vi "VFD communication.vi"() -> ()   [LabVIEW 2018]
uses:
  <vilib>/Utility/miscctls.llb/LVRectTypeDef.ctl
  <vilib>/Modbus/subvis/Modbus API/Modbus API.lvclass/Modbus API.ctl
  <vilib>/Modbus/subvis/Transmission Data Unit (ADU)/Transmission Data Unit/Transmission Data Unit.lvclass/Transmission Data Unit.ctl
  <vilib>/Modbus/master/Data Access/Unit ID/Set Unit ID Property.vi
  <vilib>/Modbus/subvis/Transmission Data Unit (ADU)/Transmission Data Unit/Data Access/Unit ID/Write Unit ID.vi
  <vilib>/Modbus/subvis/Modbus API/Read Transmission Data Unit.vi
  <vilib>/Modbus/subvis/Modbus API/Write Transmission Data Unit.vi
  <vilib>/Modbus/master/Modbus Master.lvclass
  C:/Program Files/National Instruments/LabVIEW 2018/vi.lib/Modbus/subvis/Modbus API/Modbus API.lvclass
  <vilib>/Modbus/master/Create Master Instance (TCP).vi
  <vilib>/Modbus/subvis/Transmission Data Unit (ADU)/Transmission Data Unit/Transmission Data Unit.lvclass
  <vilib>/rvi/interface/nirviOpenFPGA/nirviOpenFPGA.xnode
  <vilib>/rvi/interface/nirviMethod/nirviMethod.xnode
  <vilib>/FPGAPlugInAG/Dynamic/niLvFpga_Reset_Dynamic.vi
  <vilib>/FPGAPlugInAG/Dynamic/niLvFpga_Run_Dynamic.vi
  <vilib>/rvi/interface/nirviCloseFPGA/nirviCloseFPGA.xnode
  <vilib>/FPGAPlugInAG/Dynamic/niLvFpga_Abort_Dynamic.vi
  <vilib>/FPGAPlugInAG/Dynamic/niLvFpga_Close_Dynamic.vi
  FPGA Bitfiles/Main_FPGA_V3.lvbitx
  Main_FPGA.vi
  <vilib>/FPGAPlugInAG/cRIO-9082/niLvFpga_Open_cRIO-9082.vi
  <vilib>/rvi/interface/common/dynamic/niFpgaDynamicAddResources.vi
  <vilib>/eio/EIONode/EIONode.xnode
  <vilib>/rvi/eio/common/nirviEmuTemplateMethod_errors.vi
panel:
  in  "SPEED RPM":dbl format="%#_13g"
  in  "Brake_H":bool
  in  "Reset_H":bool
  in  "Control_H":bool
  in  "SPEED":bool
  in  "TORQUE":bool
  in  "Stop Button":bool
  out "x/y":dbl
  in  "Torque_Reference_LR 2":dbl(slide) caption="Torque \nReference" scale=-2000.0..2000.0
  out "appended array":u16[](array[numeric])
  out "*(type *) &x":i16
  out "register values":u16[](array[numeric])
  out "RPM":dbl[](array[numeric])
  in  "stop":bool
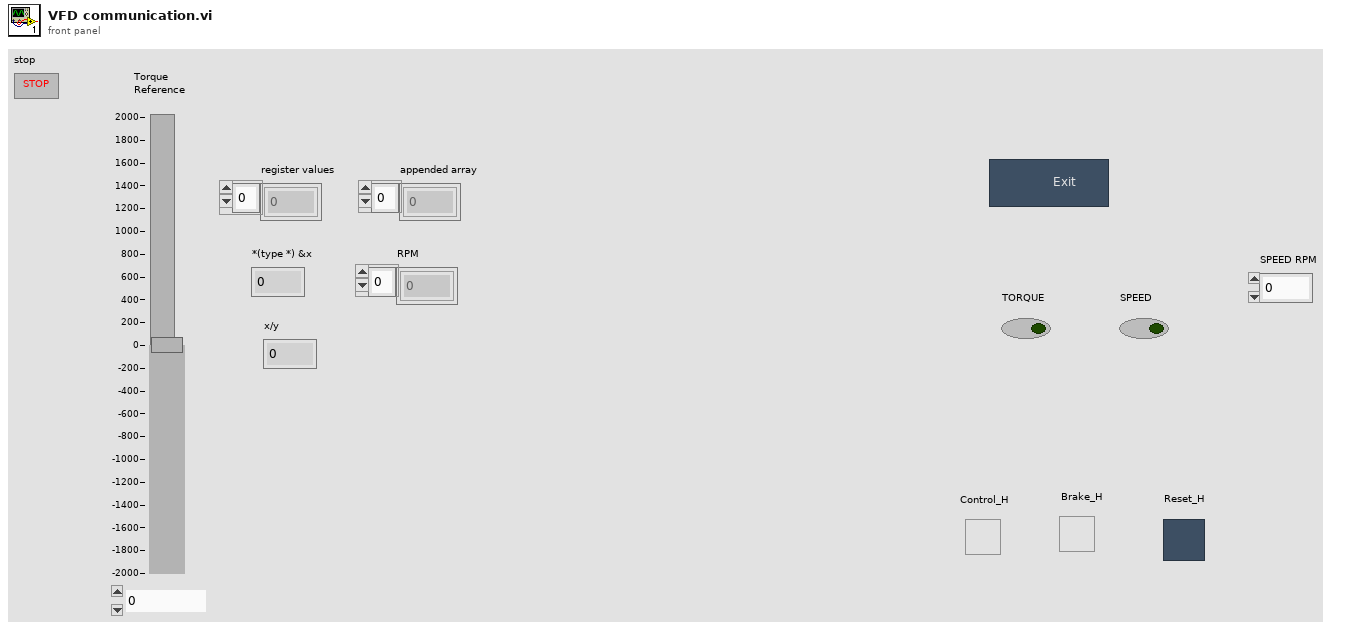
[diagram p1: front panel]
types:
  T1 = enum32{"Invalid", "Standard", "Closed", "Hidden", "Minimized", "Maximized"}
  T2 = enum32{"invalid app kind", "Development System", "Run Time System", "Student Edition", "Embedded LabVIEW", "Evaluation", "Custom"}
  T3 = typedef "LVRectTypeDef.ctl" = cluster{"Left":i16, "Top":i16, "Right":i16, "Bottom":i16}
  T4 = cluster{"Core":cluster{"Current VI Reference":refnum<vi>, "Close Panel on Exit?":bool}, "Your Boolean data":bool, "SPEED":u16[]}
  T5 = cluster{"Current VI Reference":refnum<vi>, "Close Panel on Exit?":bool}
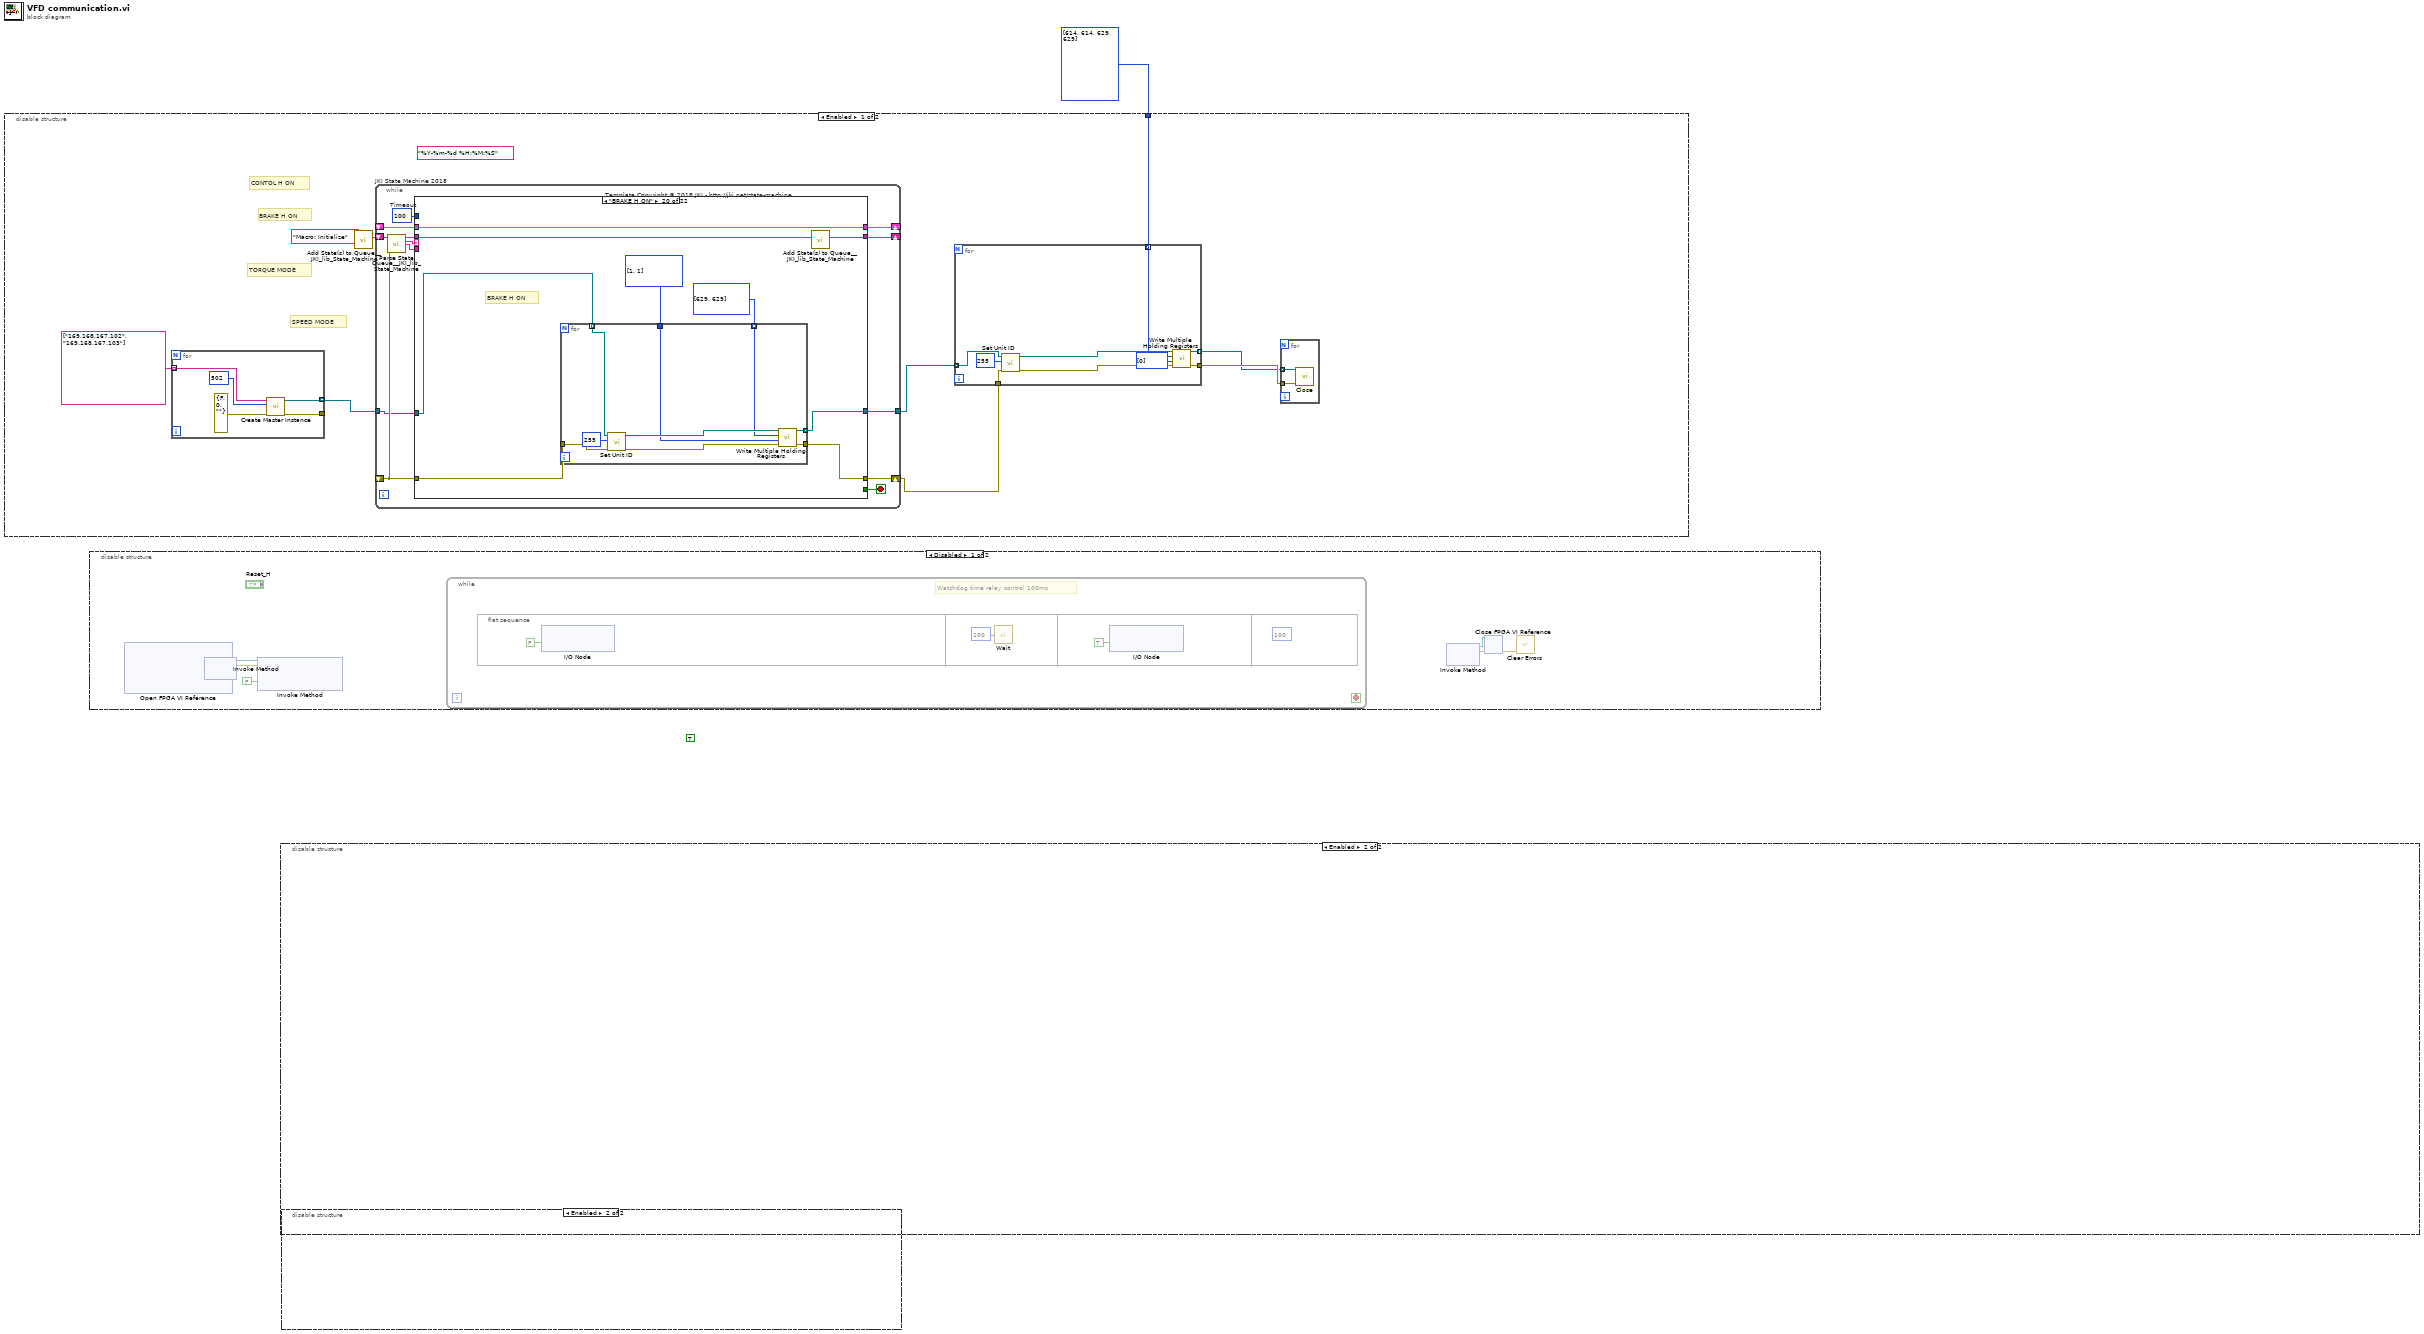
[diagram p0: block diagram]
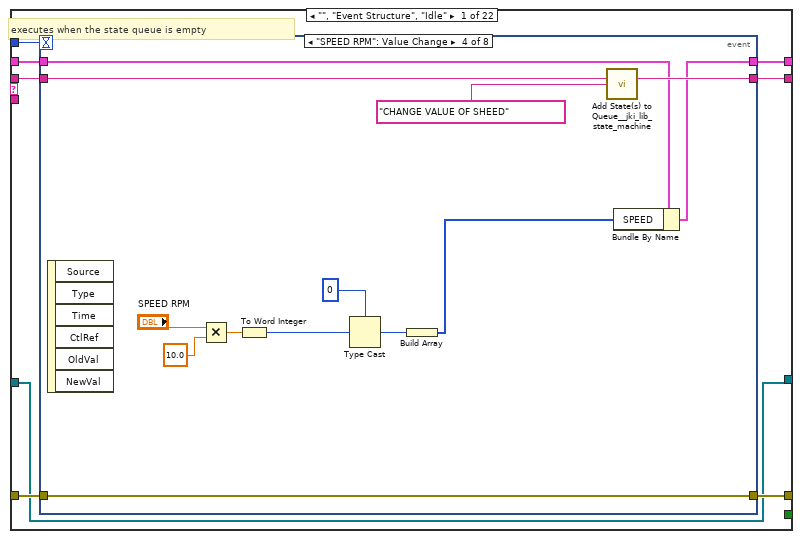
[diagram p3: hidden frame]
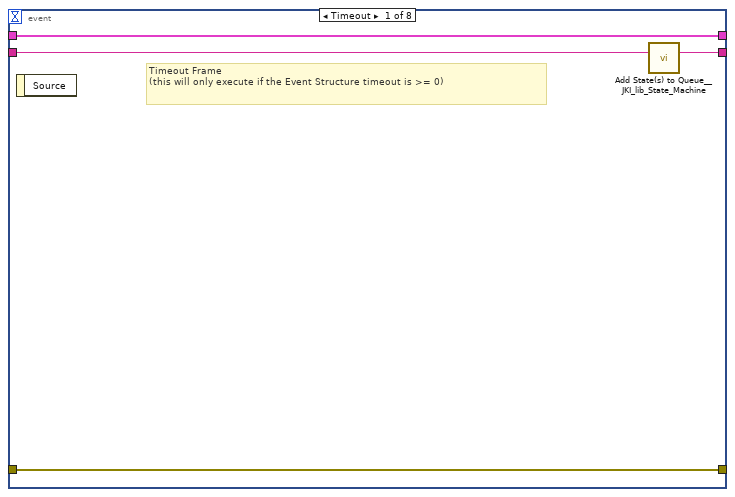
[diagram p4: hidden frame]
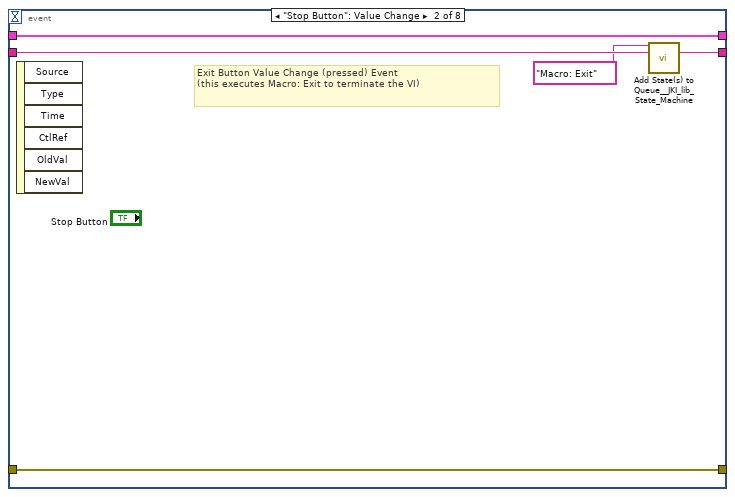
[diagram p5: hidden frame]
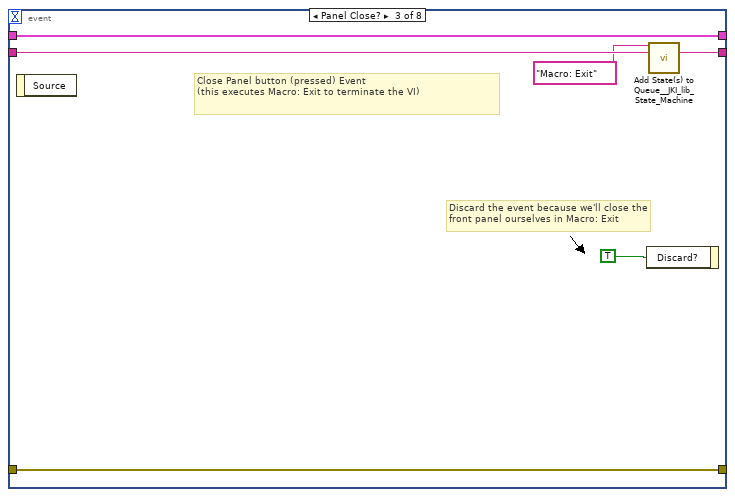
[diagram p6: hidden frame]
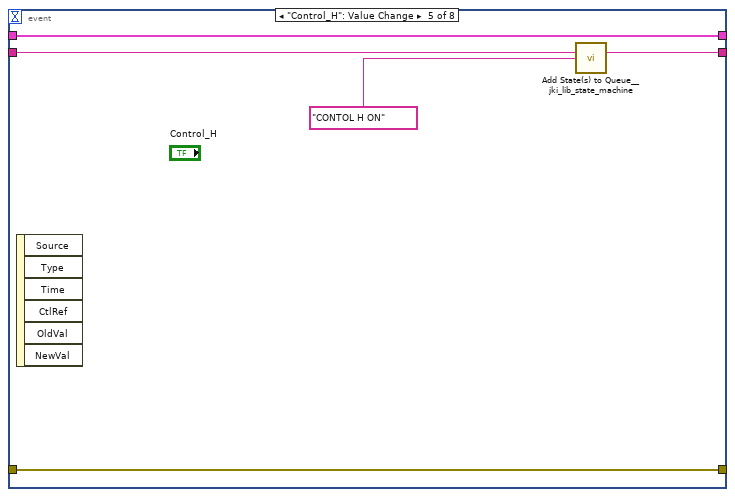
[diagram p7: hidden frame]
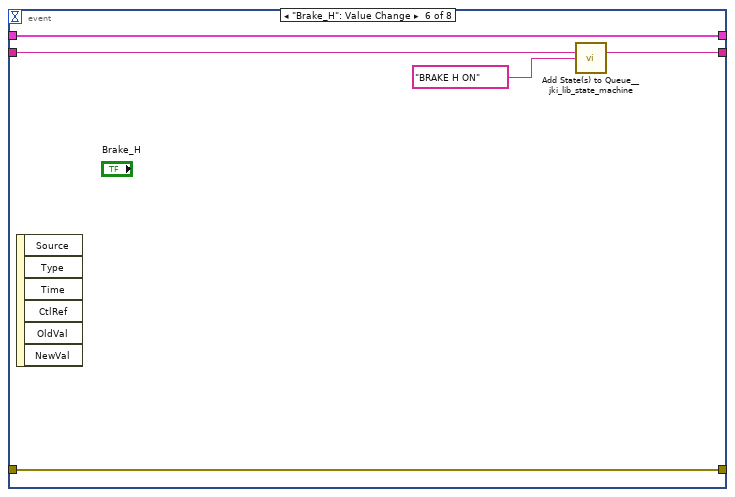
[diagram p8: hidden frame]
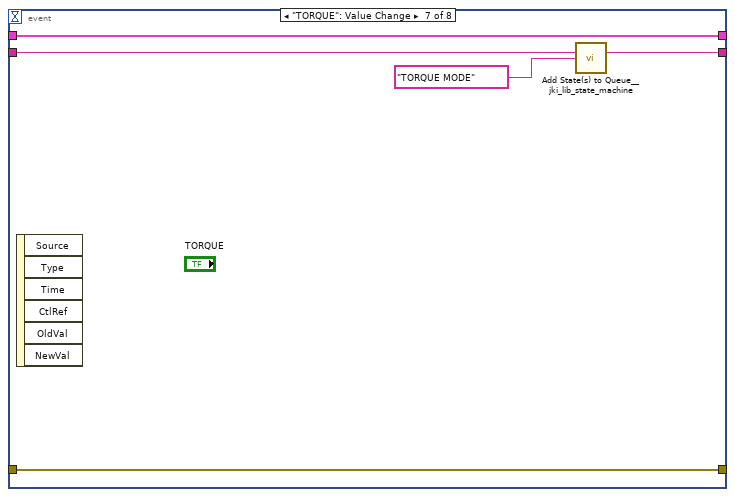
[diagram p9: hidden frame]
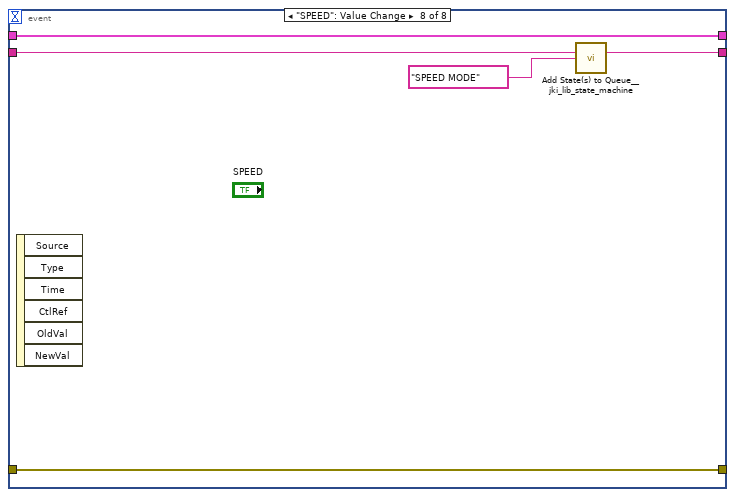
[diagram p10: hidden frame]
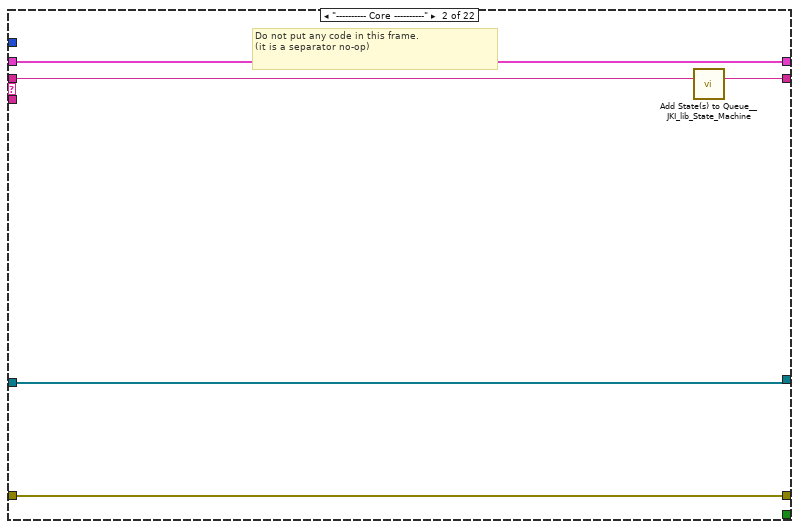
[diagram p11: hidden frame]
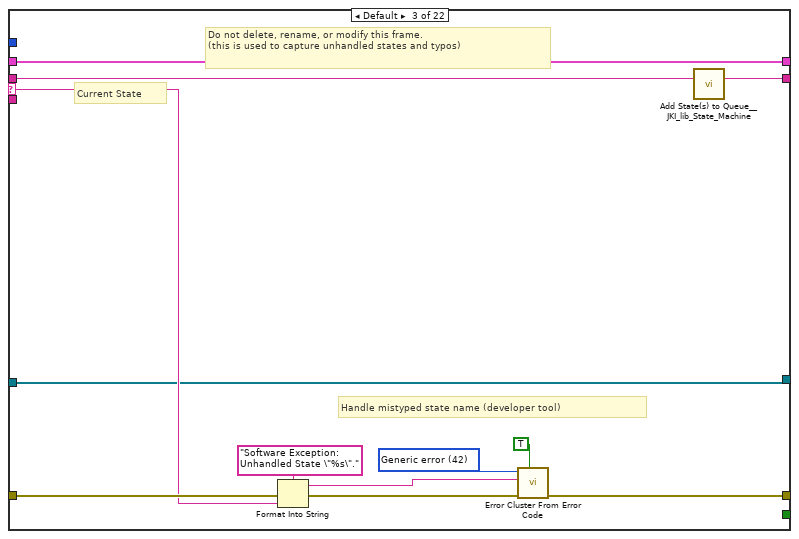
[diagram p12: hidden frame]
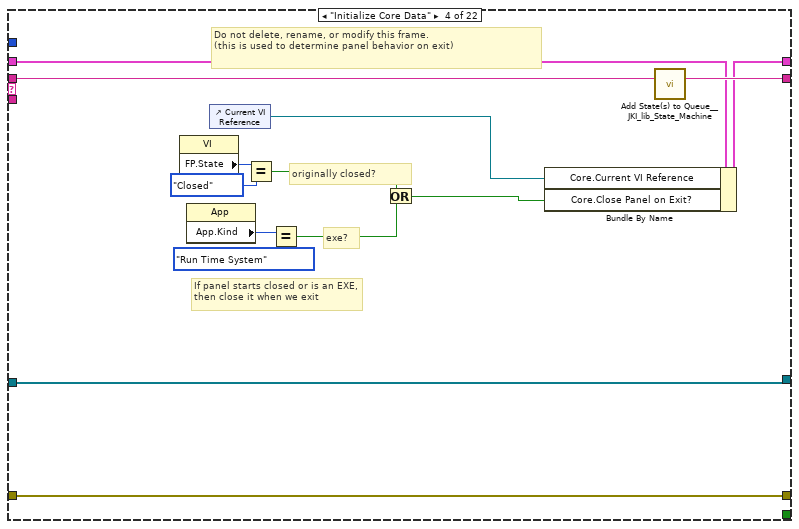
[diagram p13: hidden frame]
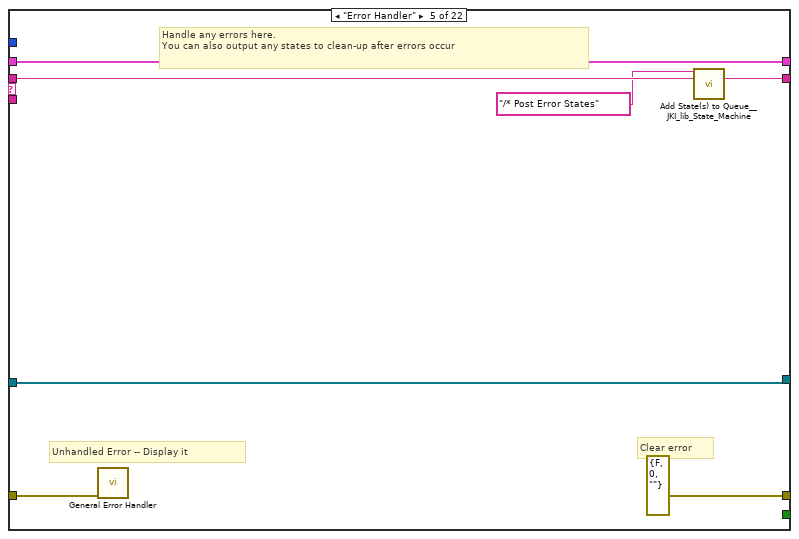
[diagram p14: hidden frame]
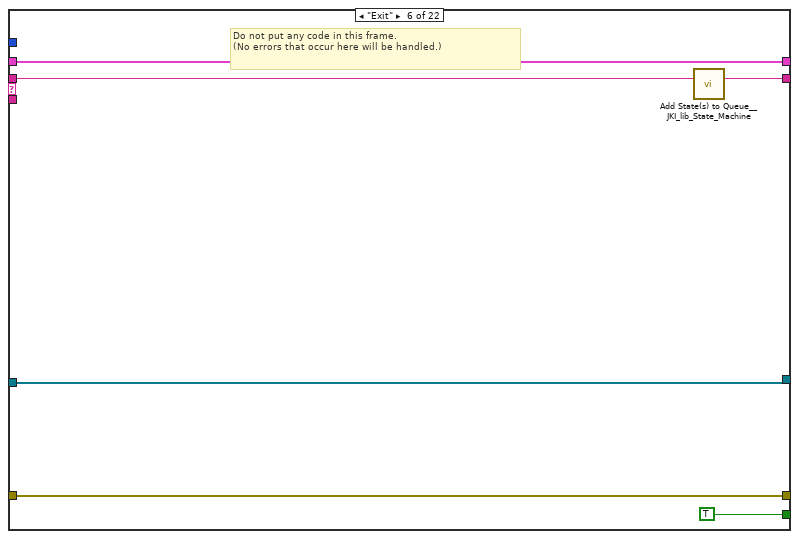
[diagram p15: hidden frame]
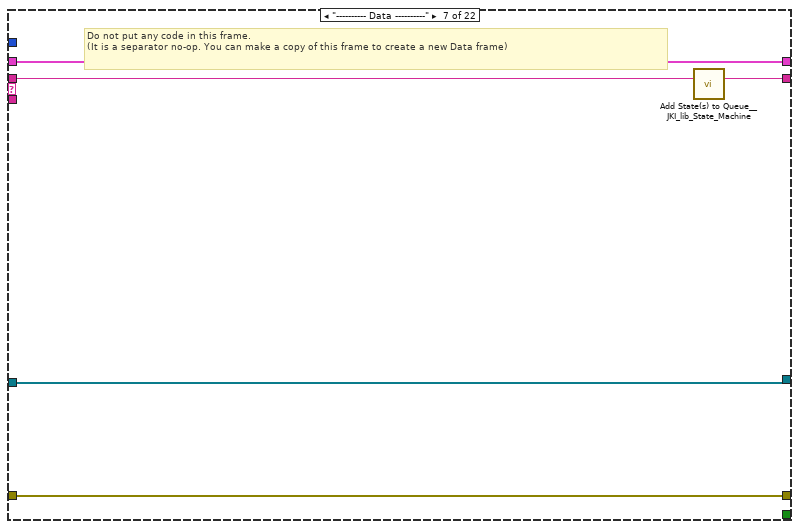
[diagram p16: hidden frame]
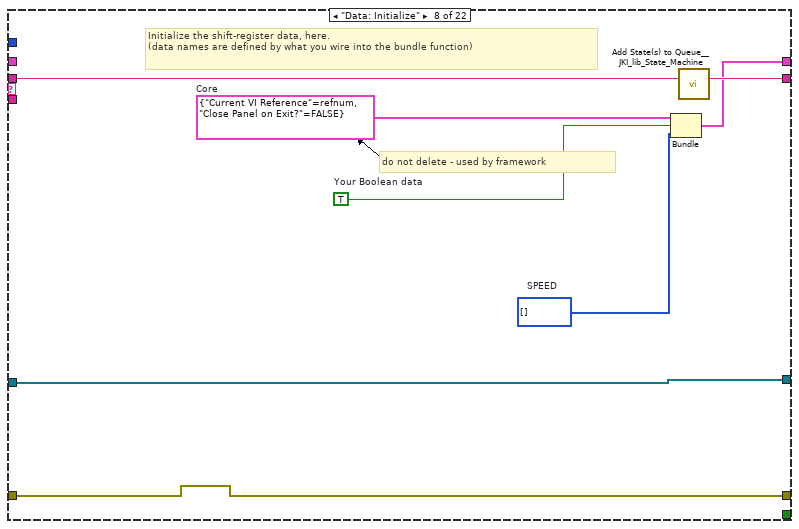
[diagram p17: hidden frame]
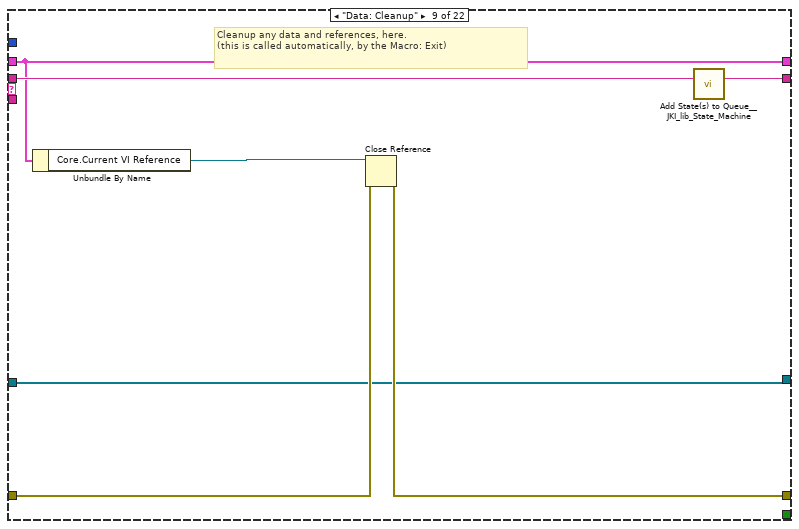
[diagram p18: hidden frame]
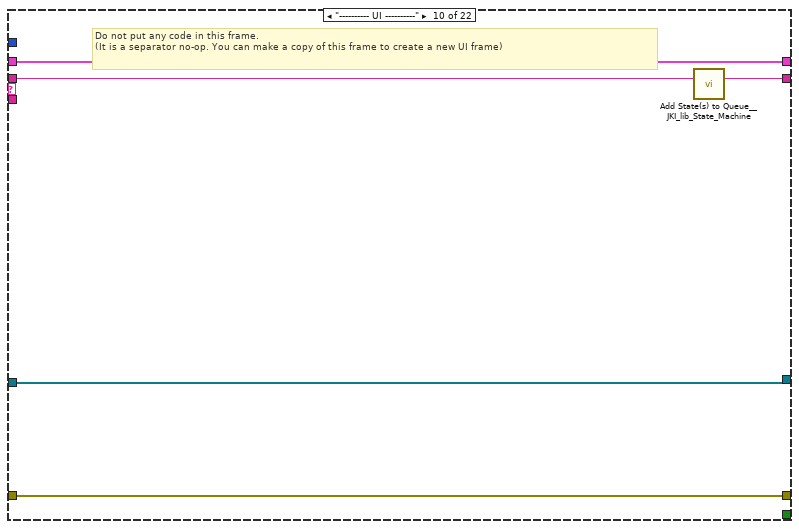
[diagram p19: hidden frame]
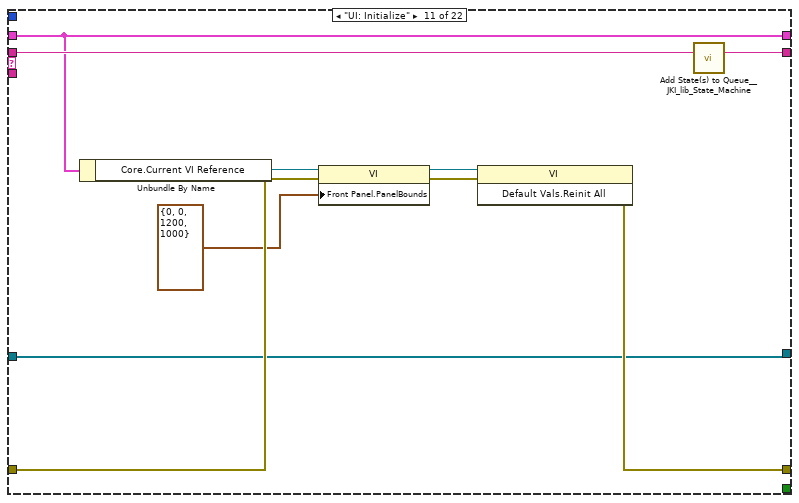
[diagram p20: hidden frame]
diagram:
  (unwired) TRUE ("Mod6/Watchdog Ready")
  n1 = disable-structure shown="Enabled" {
    disable-tunnel: u16[] [614, 614, 629, 629] ("holding register values") -> [w2 _]
    frame Enabled {
      (unwired) "%Y-%m-%d %H:%M:%S" ("time format string (%c)")
      # "SPEED MODE"
      # "TORQUE MODE"
      # "BRAKE H ON"
      # "CONTOL H ON"
      n2 = for {
        tunnel: [w24] -> _
        tunnel: string[] ["169.168.167.102", "169.168.167.103"] -> [w23] mode=indexing
        tunnel: [w22] -> w7 mode=indexing
        n3 = call-poly <vilib>:"Create Master Instance.vi"("error in (no error)"=errorcluster {"status"=FALSE, "code"=0, "source"=""}, "port (502)"=u16 502, "address"=w23) -> ("error out"=w24:errorcluster, "TCP master instance"=w22:refnum<class "Modbus Master.lvclass">)  [unwired: 7 in]
      }
      n4 = call <vilib>:"Add State(s) to Queue__JKI_lib_State_Machine.vi"("State(s) in (\"\")"="Macro: Initialize") -> ("States Out"=w10:string)  [unwired: 14 in]
      n5 = while "JKI State Machine 2018" {
        shift-right: [w32] -> _
        shift-left: _ -> [w31]
        shift-right: [w35] -> w5
        shift-left: _ -> [w29]
        shift-right: [w34] -> _
        shift-left: w10 -> [w36]
        tunnel: w7 -> [w28]
        tunnel: [w27] -> w6
        stop <- w33 stop-if-true
        w30 = 100  # Timeout
        # "Template Copyright © 2018 JKI - http://jki.net/state-machine"
        n6 = call <vilib>:"Parse State Queue__JKI_lib_State_Machine.vi"("State Queue"=w36, "Error In (no error)"=w29) -> ("Remaining States"=w38:string, "Current State"=w39:string, "Arguments"=w37:string)  [unwired: 11 in]
        n7 = case shown="\"BRAKE H ON\"" w39 {
          selector: w39 -> [_ _ w102 _ _ _ _ _ _ _ _ _ _ _ _ _ _ _ _ _ _ _]
          tunnel: w38 -> [w47 w100 w106 w126 w133 w139 w144 w152 w159 w164 w174 w181 w193 w263 w269 w280 w285 w294 w312 w330 w348 w366]
          tunnel: w37 -> [_ _ _ _ _ _ _ _ _ _ _ w176 w187 _ _ _ _ _ _ _ _ _]
          tunnel: w31 -> [w45 w97 w104 w119 w130 w137 w141 _ w154 w161 w172 w179 w189 w260 w266 w277 w282 w292 w310 w328 w346 w364]
          tunnel: [w44 w98 w108 w123 errorcluster {"status"=FALSE, "code"=0, "source"=""} ("error out") w136 w142 w147 w155 w162 w166 w177 w190 w261 w267 w278 w283 w290 w308 w326 w344 w362] -> w35
          tunnel: w29 -> [w43 w98 w107 w123 w129 w136 w142 w147 w156 w162 w170 w178 w191 w261 w267 w278 w283 w291 w309 w327 w345 w363]
          tunnel: [w46 w99 w105 w125 w132 w138 w143 w151 w158 w163 w173 w180 w192 w262 w268 w279 w284 w293 w311 w329 w347 w365] -> w34
          tunnel: [_ _ _ _ _ TRUE _ _ _ _ _ _ _ _ _ _ _ _ _ _ _ _] -> w33
          tunnel: [w42 w97 w104 w124 w130 w137 w141 w150 w154 w161 w172 w179 w189 w260 w266 w277 w282 w292 w310 w328 w346 w364] -> w32
          tunnel: w30 -> [w41 _ _ _ _ _ _ _ _ _ _ _ _ _ _ _ _ _ _ _ _ _]
          tunnel: [w40 w96 w101 w113 w127 w134 w140 w146 w153 w160 w165 w175 w186 w259 w264 w270 w281 w288 w304 w322 w340 w358] -> w27
          tunnel: w28 -> [w40 w96 w101 w113 w127 w134 w140 w146 w153 w160 w165 w175 w186 w259 w264 w270 w281 w289 w307 w325 w343 w361]
          frame "", "Event Structure", "Idle" {
            # "executes when the state queue is empty"
            n8 = event shown="[3] \"SPEED RPM\": Value Change" {
              selector: _ -> [_ _ _ _ _ _ _ _]
              dyn-events: _ -> [_ _ _ _ _ _ _ _]
              timeout: w41 -> [_ _ _ _ _ _ _ _]
              tunnel: w47 -> [w51 w56 w62 w73 w77 w82 w87 w92]
              tunnel: [w50 w55 w61 w74 w78 w83 w88 w93] -> w46
              tunnel: w45 -> [w48 w53 w59 w65 w79 w84 w89 w94]
              tunnel: [w49 w54 w60 w75 w80 w85 w90 w95] -> w44
              tunnel: w43 -> [w49 w54 w60 w75 w80 w85 w90 w95]
              tunnel: [w48 w53 w59 w63 w79 w84 w89 w94] -> w42
              event Timeout {
                # "Timeout Frame\n(this will only execute if the Event Structure timeout is >= 0)"
                n9 = event-data() -> ()  [unwired: 1 in, 1 out]
                n10 = call <vilib>:"Add State(s) to Queue__JKI_lib_State_Machine.vi"("State(s) in (\"\")"=w51) -> ("States Out"=w50:string)  [unwired: 14 in]
              }
              event "Stop Button": Value Change {
                # "Exit Button Value Change (pressed) Event\n(this executes Macro: Exit to terminate the VI)"
                n11 = event-data() -> ()  [unwired: 1 in, 6 out]
                n12 = call <vilib>:"Add State(s) to Queue__JKI_lib_State_Machine.vi"("State(s) in Front (\"\")"="Macro: Exit", "State(s) in (\"\")"=w56) -> ("States Out"=w55:string)  [unwired: 13 in]
              }
              event Panel Close? {
                # "Discard the event because we'll close the front panel ourselves in Macro: Exit"
                # "Close Panel button (pressed) Event\n(this executes Macro: Exit to terminate the VI)"
                n13 = event-data() -> ()  [unwired: 1 in, 1 out]
                n14 = event-data("Discard?"=TRUE) -> ()  [unwired: 1 in, 1 out]
                n15 = call <vilib>:"Add State(s) to Queue__JKI_lib_State_Machine.vi"("State(s) in Front (\"\")"="Macro: Exit", "State(s) in (\"\")"=w62) -> ("States Out"=w61:string)  [unwired: 13 in]
              }
              event "SPEED RPM": Value Change {
                n16 = event-data() -> ()  [unwired: 1 in, 6 out]
                n17 = Multiply(x="SPEED RPM", y=10.0) -> (x*y=w68:dbl)
                n18 = To Word Integer(number=w68) -> (16bit integer=w70:i16)
                n19 = Type Cast(type=u16 0, x=w70) -> (*(type *) &x=w69:u16)
                n20 = Build Array(w69) -> (w64:u16[])
                n21 = call <vilib>:"Add State(s) to Queue__jki_lib_state_machine.vi"("State(s) in (\"\")"=w73, "State(s) at Back (\"\")"="CHANGE VALUE OF SHEED" ("State(s) at Back (\"\")")) -> ("States Out"=w74:string)  [unwired: 13 in]
                n22 = Bundle By Name(cluster=w65, "SPEED"=w64) -> (w63:T4)
              }
              event "Control_H": Value Change {
                n23 = event-data() -> ()  [unwired: 1 in, 6 out]
                n24 = call <vilib>:"Add State(s) to Queue__jki_lib_state_machine.vi"("State(s) in (\"\")"=w77, "State(s) at Back (\"\")"="CONTOL H ON" ("State(s) at Back (\"\")")) -> ("States Out"=w78:string)  [unwired: 13 in]
              }
              event "Brake_H": Value Change {
                n25 = event-data() -> ()  [unwired: 1 in, 6 out]
                n26 = call <vilib>:"Add State(s) to Queue__jki_lib_state_machine.vi"("State(s) in (\"\")"=w82, "State(s) at Back (\"\")"="BRAKE H ON" ("State(s) at Back (\"\")")) -> ("States Out"=w83:string)  [unwired: 13 in]
              }
              event "TORQUE": Value Change {
                n27 = event-data() -> ()  [unwired: 1 in, 6 out]
                n28 = call <vilib>:"Add State(s) to Queue__jki_lib_state_machine.vi"("State(s) in (\"\")"=w87, "State(s) at Back (\"\")"="TORQUE MODE" ("State(s) at Back (\"\")")) -> ("States Out"=w88:string)  [unwired: 13 in]
              }
              event "SPEED": Value Change {
                n29 = event-data() -> ()  [unwired: 1 in, 6 out]
                n30 = call <vilib>:"Add State(s) to Queue__jki_lib_state_machine.vi"("State(s) in (\"\")"=w92, "State(s) at Back (\"\")"="SPEED MODE" ("State(s) at Back (\"\")")) -> ("States Out"=w93:string)  [unwired: 13 in]
              }
            }
          }
          frame "---------- Core ----------" {
            # "Do not put any code in this frame.\n(it is a separator no-op)"
            n31 = call <vilib>:"Add State(s) to Queue__JKI_lib_State_Machine.vi"("State(s) in (\"\")"=w100) -> ("States Out"=w99:string)  [unwired: 14 in]
          }
          frame Default {
            w111 = 42 items=["No error", "Argument error", "Memory is full", "Out of zone", "End of file", "File already open", "Generic file I/O error", "File not found", "File permission error", "Disk is full", "Duplicate path", "Too many files open", "System feature not enabled", "Resource file not found", "Cannot add resource", "Resource not found", "Image not found", "Image memory error", "Pen does not exist", "Config type invalid", "Config token not found", "Config parse error", "Config memory error", "Bad external code format", "Bad external code offset", "External code not present", "Null window", "Destroy window error", "Null menu", "Print aborted", "Bad print record", "Print driver error", "Windows error during printing", "Memory error during printing", "Print dialog error", "Generic print error", "Invalid device refnum", "Device not found", "Device parameter error", "Device unit error", "Cannot open device", "Device call aborted", "Generic error", "Cancelled by user", "Object ID too low", "Object ID too high", "Object not in heap", "Unknown heap", "Unknown object (invalid DefProc)", "Unknown object (DefProc not in table)", "Message out of range", "Invalid (null) method", "Unknown message", "Manager call not supported", "Bad address", "Network operation in progress", "Network operation timed out", "Connection is busy", "Network attribute not supported", "Network error", "Address in use", "System out of memory", "Connection aborted", "Connection refused", "Not connected", "Already connected", "Connection closed", "Initialization error (interapplication manager)", "Bad occurrence", "Wait on unbound occurrence handler", "Occurrence queue overflow", "Datalog type conflict", "Unused", "Unrecognized type (interapplication manager)", "Memory corrupt", "Failed to make temporary DLL", "Old CIN version", "Drag socket not found", "Failed to load drop-object", "Failed to register OLE object", "Failed to release OLE object", "Format specifier type mismatch", "Unknown format specifier", "Too few format specifiers", "Too many format specifiers", "Scan failed", "Newer CIN version", "Error converting to variant", "Runtime menu error", "Password tampered", "Variant attribute not found", "Incompatible variant data type", "Event data is not available", "Event Store is not present", "Occurrence is not found", "Event Queue is not created", "Event info is not available", "Refnum passed is NULL", "Error retrieving Class GUID", "Error retrieving CoClass GUID", "Error retrieving TypeLib GUID.", "Bad built application magic bytes.", "Specific driver is different from the specific driver associated with the Logical Name.", "There is no session opened to the class driver.", "Max Error", "MAX - Error with config objects", "MAX - Error loading configuration", "MAX - Group not supported"]
            # "Current State"
            # "Do not delete, rename, or modify this frame.\n(this is used to capture unhandled states and typos)"
            # "Handle mistyped state name (developer tool)"
            n32 = Format Into String(format string="Software Exception: Unhandled State \"%s\"." ("message"), error in=w107, w102) -> (resulting string=w110:string, error out=w109:errorcluster)  [unwired: 1 in]
            n33 = call <vilib>:"Error Cluster From Error Code.vi"("show call chain? (False)"=TRUE, "error in (no error)"=w109, "error message (\"\")"=w110, "error code (0)"=w111) -> ("error out"=w108:errorcluster)  [unwired: 5 in]
            n34 = call <vilib>:"Add State(s) to Queue__JKI_lib_State_Machine.vi"("State(s) in (\"\")"=w106) -> ("States Out"=w105:string)  [unwired: 14 in]
          }
          frame "Initialize Core Data" {
            # "Do not delete, rename, or modify this frame.\n(this is used to determine panel behavior on exit)"
            # "originally closed?"
            # "exe?"
            # "If panel starts closed or is an EXE, then close it when we exit"
            n35 = property class="VI"() -> ("FP.State"=w116:T1)  [unwired: 2 in, 2 out]
            n36 = property class="App"() -> ("App.Kind"=w122:T2)  [unwired: 2 in, 2 out]
            n37 = control-ref of="Current VI Reference"() -> (w117:refnum<vi>)
            n38 = Equal?(x=w116, y=T1."Closed" ("Front Panel Window:State")) -> (x = y?=w114:bool)
            n39 = Equal?(x=w122, y=T2."Run Time System" ("Application:Kind")) -> (x = y?=w120:bool)
            n40 = Or(x=w114, y=w120) -> (x .or. y?=w118:bool)
            n41 = Bundle By Name(cluster=w119, "Core.Current VI Reference"=w117, "Core.Close Panel on Exit?"=w118) -> (w124:T4)
            n42 = call <vilib>:"Add State(s) to Queue__JKI_lib_State_Machine.vi"("State(s) in (\"\")"=w126) -> ("States Out"=w125:string)  [unwired: 14 in]
          }
          frame "Error Handler" {
            # "Unhandled Error -- Display it"
            # "Handle any errors here.\nYou can also output any states to clean-up after errors occur"
            # "Clear error"
            n43 = call <vilib>:"General Error Handler.vi"("error in (no error)"=w129) -> ()  [unwired: 10 in, 5 out]
            n44 = call <vilib>:"Add State(s) to Queue__JKI_lib_State_Machine.vi"("State(s) in Front (\"\")"="/* Post Error States", "State(s) in (\"\")"=w133) -> ("States Out"=w132:string)  [unwired: 13 in]
          }
          frame "Exit" {
            # "Do not put any code in this frame.\n(No errors that occur here will be handled.)"
            n45 = call <vilib>:"Add State(s) to Queue__JKI_lib_State_Machine.vi"("State(s) in (\"\")"=w139) -> ("States Out"=w138:string)  [unwired: 14 in]
          }
          frame "---------- Data ----------" {
            # "Do not put any code in this frame.\n(It is a separator no-op. You can make a copy of this frame to create a new Data frame)"
            n46 = call <vilib>:"Add State(s) to Queue__JKI_lib_State_Machine.vi"("State(s) in (\"\")"=w144) -> ("States Out"=w143:string)  [unwired: 14 in]
          }
          frame "Data: Initialize" {
            w145 = u16[] []  # SPEED
            w148 = T5 {"Current VI Reference"=refnum, "Close Panel on Exit?"=FALSE}  # Core
            w149 = TRUE  # Your Boolean data
            # "do not delete - used by framework"
            # "Initialize the shift-register data, here.\n(data names are defined by what you wire into the bundle function)"
            n47 = Bundle("Core"=w148, "Your Boolean data"=w149, "SPEED"=w145) -> (w150:T4)  [unwired: 1 in]
            n48 = call <vilib>:"Add State(s) to Queue__JKI_lib_State_Machine.vi"("State(s) in (\"\")"=w152) -> ("States Out"=w151:string)  [unwired: 14 in]
          }
          frame "Data: Cleanup" {
            # "Cleanup any data and references, here.\n(this is called automatically, by the Macro: Exit)"
            n49 = Unbundle By Name(w154) -> ("Core.Current VI Reference"=w157:refnum<vi>)
            n50 = Close Reference(reference=w157, error in (no error)=w156) -> (error out=w155:errorcluster)
            n51 = call <vilib>:"Add State(s) to Queue__JKI_lib_State_Machine.vi"("State(s) in (\"\")"=w159) -> ("States Out"=w158:string)  [unwired: 14 in]
          }
          frame "---------- UI ----------" {
            # "Do not put any code in this frame.\n(It is a separator no-op. You can make a copy of this frame to create a new UI frame)"
            n52 = call <vilib>:"Add State(s) to Queue__JKI_lib_State_Machine.vi"("State(s) in (\"\")"=w164) -> ("States Out"=w163:string)  [unwired: 14 in]
          }
          frame "UI: Initialize" {
            n53 = Unbundle By Name(w172) -> ("Core.Current VI Reference"=w171:refnum<vi>)
            n54 = property class="VI"(reference=w171, error in=w170, "Front Panel.PanelBounds"=T3 {"Left"=0, "Top"=0, "Right"=1200, "Bottom"=1000} ("Front Panel Window:Panel Bounds")) -> (reference out=w168:refnum<vi>, error out=w167:errorcluster)
            n55 = invoke class="VI" method="Default Vals.Reinit All"(reference=w168, error in=w167) -> (error out=w166:errorcluster)  [unwired: 1 in, 2 out]
            n56 = call <vilib>:"Add State(s) to Queue__JKI_lib_State_Machine.vi"("State(s) in (\"\")"=w174) -> ("States Out"=w173:string)  [unwired: 14 in]
          }
          frame "UI: Cursor Set" {
            # "Argument"
            # "Set and Unset Cursor Busy.\n(Usage: \"UI: Cursor Set >> Busy|Idle\")"
            n57 = case shown="\"Idle\", Default" w176 {
              tunnel: w178 -> [w183 w185]
              tunnel: [w182 w184] -> w177
              frame "Idle", Default {
                n58 = call <vilib>:"Unset Busy.vi"("error in (no error)"=w183) -> ("error out"=w182:errorcluster)  [unwired: 10 in]
              }
              frame "Busy" {
                n59 = call <vilib>:"Set Busy.vi"("error in (no error)"=w185) -> ("error out"=w184:errorcluster)  [unwired: 9 in, 1 out]
              }
            }
            n60 = call <vilib>:"Add State(s) to Queue__JKI_lib_State_Machine.vi"("State(s) in (\"\")"=w181) -> ("States Out"=w180:string)  [unwired: 14 in]
          }
          frame "UI: Front Panel State" {
            # "Argument"
            # "Set Front Panel Open or Closed\n(Usage: \"UI: Front Panel State >> Open|Close\")"
            n61 = Unbundle By Name(w189) -> ("Core.Current VI Reference"=w188:refnum<vi>)
            n62 = case shown="\"Minimize\", \"Minimized\"" w187 {
              tunnel: w191 -> [w199 w214 w225 w238 w251]
              tunnel: [w201 w215 w227 w240 w253] -> w190
              tunnel: w188 -> [w200 w212 w226 w239 w252]
              frame "Open", "Standard", Default {
                w194 = T1."Standard" ("State")
                n63 = property class="VI"(reference=w200, error in=w199) -> (reference out=w197:refnum<vi>, error out=w198:errorcluster, "FP.State"=w196:T1)
                n64 = Not Equal?(x=w196, y=w194) -> (x != y?=w195:bool)
                n65 = case shown="True" w195 {
                  tunnel: [w205 w207] -> w201
                  tunnel: w198 -> [w204 w207]
                  tunnel: w197 -> [w203 _]
                  tunnel: w194 -> [w202 _]
                  frame True {
                    n66 = invoke class="VI" method="FP.Open"(reference=w203, error in=w204, "Activate"=TRUE, "State"=w202) -> (error out=w205:errorcluster)  [unwired: 1 in, 4 out]
                  }
                  frame False {
                  }
                }
              }
              frame "Close", "Closed" {
                n67 = property class="VI"(reference=w212, error in=w214) -> (reference out=w211:refnum<vi>, error out=w213:errorcluster, "FP.State"=w209:T1)
                n68 = Not Equal?(x=w209, y=T1."Closed" ("Front Panel Window:State")) -> (x != y?=w208:bool)
                n69 = case shown="True" w208 {
                  tunnel: [w216 w219] -> w215
                  tunnel: w213 -> [w216 w218]
                  tunnel: w211 -> [_ w217]
                  frame False {
                  }
                  frame True {
                    n70 = invoke class="VI" method="FP.Close"(reference=w217, error in=w218) -> (error out=w219:errorcluster)  [unwired: 1 in, 2 out]
                  }
                }
              }
              frame "Hidden", "Hide" {
                w220 = T1."Hidden" ("State")
                n71 = property class="VI"(reference=w226, error in=w225) -> (reference out=w223:refnum<vi>, error out=w224:errorcluster, "FP.State"=w222:T1)
                n72 = Not Equal?(x=w222, y=w220) -> (x != y?=w221:bool)
                n73 = case shown="True" w221 {
                  tunnel: [w231 w232] -> w227
                  tunnel: w224 -> [w230 w232]
                  tunnel: w223 -> [w229 _]
                  tunnel: w220 -> [w228 _]
                  frame True {
                    n74 = invoke class="VI" method="FP.Open"(reference=w229, error in=w230, "State"=w228) -> (error out=w231:errorcluster)  [unwired: 2 in, 4 out]
                  }
                  frame False {
                  }
                }
              }
              frame "Minimize", "Minimized" {
                w233 = T1."Minimized" ("State")
                n75 = property class="VI"(reference=w239, error in=w238) -> (reference out=w236:refnum<vi>, error out=w237:errorcluster, "FP.State"=w235:T1)
                n76 = Not Equal?(x=w235, y=w233) -> (x != y?=w234:bool)
                n77 = case shown="True" w234 {
                  tunnel: [w244 w245] -> w240
                  tunnel: w237 -> [w243 w245]
                  tunnel: w236 -> [w242 _]
                  tunnel: w233 -> [w241 _]
                  frame True {
                    n78 = invoke class="VI" method="FP.Open"(reference=w242, error in=w243, "State"=w241) -> (error out=w244:errorcluster)  [unwired: 2 in, 4 out]
                  }
                  frame False {
                  }
                }
              }
              frame "Maximize", "Maximized" {
                w246 = T1."Maximized" ("State")
                n79 = property class="VI"(reference=w252, error in=w251) -> (reference out=w249:refnum<vi>, error out=w250:errorcluster, "FP.State"=w248:T1)
                n80 = Not Equal?(x=w248, y=w246) -> (x != y?=w247:bool)
                n81 = case shown="True" w247 {
                  tunnel: [w257 w258] -> w253
                  tunnel: w250 -> [w256 w258]
                  tunnel: w249 -> [w255 _]
                  tunnel: w246 -> [w254 _]
                  frame True {
                    n82 = invoke class="VI" method="FP.Open"(reference=w255, error in=w256, "State"=w254) -> (error out=w257:errorcluster)  [unwired: 2 in, 4 out]
                  }
                  frame False {
                  }
                }
              }
            }
            n83 = call <vilib>:"Add State(s) to Queue__JKI_lib_State_Machine.vi"("State(s) in (\"\")"=w193) -> ("States Out"=w192:string)  [unwired: 14 in]
          }
          frame "---------- Macro ----------" {
            # "Do not put any code in this frame.\n(It is a separator no-op. You can make a copy of this frame to create a new Macro frame)"
            n84 = call <vilib>:"Add State(s) to Queue__JKI_lib_State_Machine.vi"("State(s) in (\"\")"=w263) -> ("States Out"=w262:string)  [unwired: 14 in]
          }
          frame "Macro: Initialize" {
            w265 = "Data: Initialize\nInitialize Core Data\nUI: Initialize\nUI: Front Panel State >> Open"  # Data: Initialize Initialize Core Data UI: Initialize UI: Front Panel State >> Open
            # "Initialization Macro\n(This is called once, when the VI starts)"
            n85 = call <vilib>:"Add State(s) to Queue__JKI_lib_State_Machine.vi"("State(s) in Front (\"\")"=w265, "State(s) in (\"\")"=w269) -> ("States Out"=w268:string)  [unwired: 13 in]
          }
          frame "Macro: Exit" {
            # "Exit Macro\n(This is called once, when the VI exits)"
            n86 = Unbundle By Name(w277) -> ("Core.Close Panel on Exit?"=w276:bool)
            n87 = Select(t="UI: Front Panel State >> Close", s=w276, f="") -> (s? t:f=w273:string)
            n88 = call <vilib>:"Add State(s) to Queue__JKI_lib_State_Machine.vi"("State(s) in (\"\")"=w273, "State(s) at Back (\"\")"="Data: Cleanup\nExit") -> ("States Out"=w271:string)  [unwired: 13 in]
            n89 = call <vilib>:"Add State(s) to Queue__JKI_lib_State_Machine.vi"("State(s) in Front (\"\")"=w271, "State(s) in (\"\")"=w280) -> ("States Out"=w279:string)  [unwired: 13 in]
          }
          frame "---------- New Category ----------" {
            # "Template Separator\n(You can make a copy of, or modify, this frame)"
            n90 = call <vilib>:"Add State(s) to Queue__JKI_lib_State_Machine.vi"("State(s) in (\"\")"=w285) -> ("States Out"=w284:string)  [unwired: 14 in]
          }
          frame "CHANGE VALUE OF SHEED" {
            w287 = u16[] [121, 121]  # address
            n91 = Unbundle By Name(w292) -> ("SPEED"=w286:u16[])
            n92 = for {
              tunnel: w291 -> [w298]
              tunnel: w289 -> [w300] mode=indexing
              tunnel: [w303] -> w288 mode=indexing
              tunnel: [w302] -> w290
              tunnel: w287 -> [w296] mode=indexing
              tunnel: w286 -> [w295]
              n93 = call <vilib>:"Set Unit ID.vi"("error in (no error)"=w298, "unit ID"=u8 255, "Modbus master in"=w300) -> ("error out"=w297:errorcluster, "Modbus master out"=w299:refnum<class "Modbus Master.lvclass">)  [unwired: 7 in]
              n94 = call-dynamic "Write Multiple Holding Registers.vi"("error in (no error)"=w297, "holding register values"=w295, "starting address"=w296, "Modbus master in"=w299) -> ("error out"=w302:errorcluster, "Modbus master out"=w303:refnum<class "Modbus Master.lvclass">)  [unwired: 6 in]
            }
            n95 = call <vilib>:"Add State(s) to Queue__JKI_lib_State_Machine.vi"("State(s) in (\"\")"=w294) -> ("States Out"=w293:string)  [unwired: 14 in]
          }
          frame "CONTOL H ON" {
            # "CONTOL H ON"
            n96 = for {
              tunnel: w307 -> [w315] mode=indexing
              tunnel: w309 -> [w317]
              tunnel: [w321] -> w304 mode=indexing
              tunnel: [w320] -> w308
              tunnel: u16[] [1, 1] ("holding register values") -> [w314]
              tunnel: u16[] [614, 614] ("holding register values") -> [w313] mode=indexing
              n97 = call <vilib>:"Set Unit ID.vi"("error in (no error)"=w317, "unit ID"=u8 255, "Modbus master in"=w315) -> ("error out"=w316:errorcluster, "Modbus master out"=w318:refnum<class "Modbus Master.lvclass">)  [unwired: 7 in]
              n98 = call-dynamic "Write Multiple Holding Registers.vi"("error in (no error)"=w316, "holding register values"=w314, "starting address"=w313, "Modbus master in"=w318) -> ("error out"=w320:errorcluster, "Modbus master out"=w321:refnum<class "Modbus Master.lvclass">)  [unwired: 6 in]
            }
            n99 = call <vilib>:"Add State(s) to Queue__JKI_lib_State_Machine.vi"("State(s) in (\"\")"=w312) -> ("States Out"=w311:string)  [unwired: 14 in]
          }
          frame "BRAKE H ON" {
            # "BRAKE H ON"
            n100 = for {
              tunnel: w325 -> [w333] mode=indexing
              tunnel: w327 -> [w335]
              tunnel: [w339] -> w322 mode=indexing
              tunnel: [w338] -> w326
              tunnel: u16[] [1, 1] ("holding register values") -> [w332]
              tunnel: u16[] [629, 629] ("holding register values") -> [w331] mode=indexing
              n101 = call <vilib>:"Set Unit ID.vi"("error in (no error)"=w335, "unit ID"=u8 255, "Modbus master in"=w333) -> ("error out"=w334:errorcluster, "Modbus master out"=w336:refnum<class "Modbus Master.lvclass">)  [unwired: 7 in]
              n102 = call-dynamic "Write Multiple Holding Registers.vi"("error in (no error)"=w334, "holding register values"=w332, "starting address"=w331, "Modbus master in"=w336) -> ("error out"=w338:errorcluster, "Modbus master out"=w339:refnum<class "Modbus Master.lvclass">)  [unwired: 6 in]
            }
            n103 = call <vilib>:"Add State(s) to Queue__JKI_lib_State_Machine.vi"("State(s) in (\"\")"=w330) -> ("States Out"=w329:string)  [unwired: 14 in]
          }
          frame "TORQUE MODE" {
            # "TORQUE MODE"
            n104 = for {
              tunnel: w343 -> [w351] mode=indexing
              tunnel: w345 -> [w353]
              tunnel: [w357] -> w340 mode=indexing
              tunnel: [w356] -> w344
              tunnel: u16[] [1] ("holding register values") -> [w350]
              tunnel: u16[] [1835] ("holding register values") -> [w349] mode=indexing
              n105 = call <vilib>:"Set Unit ID.vi"("error in (no error)"=w353, "unit ID"=u8 255, "Modbus master in"=w351) -> ("error out"=w352:errorcluster, "Modbus master out"=w354:refnum<class "Modbus Master.lvclass">)  [unwired: 7 in]
              n106 = call-dynamic "Write Multiple Holding Registers.vi"("error in (no error)"=w352, "holding register values"=w350, "starting address"=w349, "Modbus master in"=w354) -> ("error out"=w356:errorcluster, "Modbus master out"=w357:refnum<class "Modbus Master.lvclass">)  [unwired: 6 in]
            }
            n107 = call <vilib>:"Add State(s) to Queue__JKI_lib_State_Machine.vi"("State(s) in (\"\")"=w348) -> ("States Out"=w347:string)  [unwired: 14 in]
          }
          frame "SPEED MODE" {
            # "SPEED MODE"
            n108 = for {
              tunnel: w361 -> [w369] mode=indexing
              tunnel: w363 -> [w371]
              tunnel: [w375] -> w358 mode=indexing
              tunnel: [w374] -> w362
              tunnel: u16[] [1] ("holding register values") -> [w368]
              tunnel: u16[] [1835] ("holding register values") -> [w367] mode=indexing
              n109 = call <vilib>:"Set Unit ID.vi"("error in (no error)"=w371, "unit ID"=u8 255, "Modbus master in"=w369) -> ("error out"=w370:errorcluster, "Modbus master out"=w372:refnum<class "Modbus Master.lvclass">)  [unwired: 7 in]
              n110 = call-dynamic "Write Multiple Holding Registers.vi"("error in (no error)"=w370, "holding register values"=w368, "starting address"=w367, "Modbus master in"=w372) -> ("error out"=w374:errorcluster, "Modbus master out"=w375:refnum<class "Modbus Master.lvclass">)  [unwired: 6 in]
            }
            n111 = call <vilib>:"Add State(s) to Queue__JKI_lib_State_Machine.vi"("State(s) in (\"\")"=w366) -> ("States Out"=w365:string)  [unwired: 14 in]
          }
        }
      }
      n112 = for {
        tunnel: w6 -> [w13] mode=indexing
        tunnel: [w19] -> w3 mode=indexing
        tunnel: [w18] -> w4
        tunnel: w2 -> [w14] mode=indexing
        tunnel: w5 -> [w12]
        n113 = call <vilib>:"Set Unit ID.vi"("error in (no error)"=w12, "unit ID"=u8 255, "Modbus master in"=w13) -> ("error out"=w15:errorcluster, "Modbus master out"=w16:refnum<class "Modbus Master.lvclass">)  [unwired: 7 in]
        n114 = call-dynamic "Write Multiple Holding Registers.vi"("error in (no error)"=w15, "holding register values"=u16[] [0], "starting address"=w14, "Modbus master in"=w16) -> ("error out"=w18:errorcluster, "Modbus master out"=w19:refnum<class "Modbus Master.lvclass">)  [unwired: 6 in]
      }
      n115 = for {
        tunnel: w4 -> [w21]
        tunnel: w3 -> [w20] mode=indexing
        n116 = call-dynamic "Close.vi"("error in (no error)"=w21, "Modbus master in"=w20) -> ()  [unwired: 9 in, 1 out]
      }
    }
    frame Disabled {
    }
  }
  n117 = disable-structure shown="Disabled" {
    frame Disabled {
      n118 = xnode "Open FPGA VI Reference"() -> ("FPGA VI Reference Out"=w383:refnum<k20>, "error out"=w382:errorcluster)  [unwired: 2 in]
      n119 = xnode "Invoke Method"("FPGA VI Reference In"=w383, "error in"=w382) -> ("FPGA VI Reference Out"=w381:refnum<k20>, "error out"=w380:errorcluster)
      n120 = xnode "Invoke Method"("FPGA VI Reference In"=w381, "error in"=w380, "Wait Until Done (F)"=FALSE) -> ()  [unwired: 2 out]
      n121 = while {
        stop <- _ stop-if-true
        # "Watchdog time relay control 100ms"
        n122 = flat-sequence {
          frame #0 {
            n123 = xnode "I/O Node"("Mod4/DO16"=FALSE) -> ()  [unwired: 1 in, 1 out]
          }
          frame #1 {
            n124 = call "Wait"("Count(mSec)"=u32 100) -> ()  [unwired: 1 out]
          }
          frame #2 {
            n125 = xnode "I/O Node"("Mod4/DO16"=TRUE) -> ()  [unwired: 1 in, 1 out]
          }
          frame #3 {
            (unwired) u32 100 ("Count(mSec)")
          }
        }
      }
      n126 = xnode "Invoke Method"() -> ("FPGA VI Reference Out"=w378:refnum<k20>, "error out"=w377:errorcluster)  [unwired: 2 in]
      n127 = xnode "Close FPGA VI Reference"("FPGA VI Reference In"=w378, "error in"=w377) -> ("error out"=w376:errorcluster)
      n128 = call <vilib>:"Clear Errors.vi"("error in (no error)"=w376) -> ()  [unwired: 5 in, 2 out]
    }
    frame Enabled {
    }
  }
  n129 = disable-structure shown="Enabled" {
    frame Disabled {
      (unwired) 0.0 ("x/y")
      w392 = u16[] [408, 408]  # address
      (unwired) u16[] [146, 146]  # address
      w398 = u16[] [146, 146]  # address
      n130 = for {
        tunnel: [w469] -> w396
        tunnel: string[] ["169.168.167.102", "169.168.167.103"] -> [w468] mode=indexing
        tunnel: [w467] -> w401 mode=indexing
        n131 = call-poly <vilib>:"Create Master Instance.vi"("error in (no error)"=errorcluster {"status"=FALSE, "code"=0, "source"=""}, "port (502)"=u16 502, "address"=w468) -> ("error out"=w469:errorcluster, "TCP master instance"=w467:refnum<class "Modbus Master.lvclass">)  [unwired: 7 in]
      }
      n132 = Divide(x="Torque_Reference_LR 2", y=20.0) -> (x/y=w387:dbl)
      "x/y" <- w387
      n133 = Multiply(x=w387, y=10.0) -> (x*y=w391:dbl)
      n134 = To Word Integer(number=w391) -> (16bit integer=w399:i16)
      n135 = Type Cast(type=u16 0, x=w399) -> (*(type *) &x=w397:u16)
      n136 = Build Array(w397) -> (w393:u16[])
      "appended array" <- w393
      n137 = disable-structure shown="Disabled" {
        disable-tunnel: w401 -> [w410 w421]
        disable-tunnel: w398 -> [w409 _]
        disable-tunnel: w396 -> [w408 w420]
        disable-tunnel: [w407 w421] -> w395
        disable-tunnel: [w406 w420] -> w394
        disable-tunnel: w393 -> [w405 _]
        frame Disabled {
          n138 = for {
            tunnel: w410 -> [w414] mode=indexing
            tunnel: w405 -> [_] mode=indexing
            tunnel: w409 -> [w419] mode=indexing
            tunnel: w408 -> [w412]
            tunnel: [w417] -> w407 mode=indexing
            tunnel: [w416] -> w406 mode=indexing
            n139 = call <vilib>:"Set Unit ID.vi"("error in (no error)"=w412, "unit ID"=u8 255, "Modbus master in"=w414) -> ("error out"=w411:errorcluster, "Modbus master out"=w413:refnum<class "Modbus Master.lvclass">)  [unwired: 7 in]
            n140 = call-dynamic "Write Multiple Holding Registers.vi"("error in (no error)"=w411, "holding register values"=u16[] [1], "starting address"=w419, "Modbus master in"=w413) -> ("error out"=w416:errorcluster, "Modbus master out"=w417:refnum<class "Modbus Master.lvclass">)  [unwired: 6 in]
          }
        }
        frame Enabled {
        }
      }
      n141 = disable-structure shown="Enabled" {
        disable-tunnel: [w423 w452] -> w404
        disable-tunnel: [w422 w453] -> w402
        disable-tunnel: w395 -> [_ w454]
        disable-tunnel: w394 -> [_ w455]
        disable-tunnel: w393 -> [_ w450]
        disable-tunnel: w392 -> [_ w451]
        frame Disabled {
          n142 = while {
            shift-right: [w427] -> w423
            shift-left: _ -> [w428]
            shift-right: [w426] -> w422
            shift-left: _ -> [w429]
            stop <- "stop" stop-if-true
            n143 = for {
              shift-right: [w444] -> w427
              shift-left: w428 -> [w448]
              tunnel: [w443] -> w426 mode=indexing
              tunnel: [w435] -> w425 mode=indexing
              tunnel: w429 -> [w433] mode=indexing
              tunnel: [w432] -> w424
              w434 = u16 301  # starting address
              w439 = i16 0  # I16
              w445 = u16 1  # NHR
              n144 = call <vilib>:"Set Unit ID.vi"("error in (no error)"=w448, "unit ID"=u8 255, "Modbus master in"=w433) -> ("error out"=w446:errorcluster, "Modbus master out"=w447:refnum<class "Modbus Master.lvclass">)  [unwired: 7 in]
              n145 = call-dynamic "Read Holding Registers.vi"("error in (no error)"=w446, "number of holding registers"=w445, "starting address"=w434, "Modbus master in"=w447) -> ("error out"=w444:errorcluster, "register values"=w442:u16[], "Modbus master out"=w443:refnum<class "Modbus Master.lvclass">)  [unwired: 5 in]
              "register values" <- w442
              n146 = Index Array(array=w442, index=0) -> (element=w440:u16)
              n147 = Type Cast(type=w439, x=w440) -> (*(type *) &x=w432:i16)
              n148 = To Double Precision Float(number=w432) -> (double precision float=w438:dbl)
              n149 = Divide(x=w438, y=10.0) -> (x/y=w436:dbl)
              n150 = Absolute Value(x=w436) -> (abs(x)=w435:dbl)
            }
            "RPM" <- w425
            "*(type *) &x" <- w424
            n151 = Wait (ms)(milliseconds to wait=u32 5) -> ()  [unwired: 1 out]
          }
        }
        frame Enabled {
          n152 = for {
            tunnel: w455 -> [w457]
            tunnel: w454 -> [w459] mode=indexing
            tunnel: [w464] -> w453 mode=indexing
            tunnel: [w463] -> w452 mode=indexing
            tunnel: w451 -> [w462] mode=indexing
            tunnel: w450 -> [w461]
            (unwired) u16[] [22] ("holding register values")
            n153 = call <vilib>:"Set Unit ID.vi"("error in (no error)"=w457, "unit ID"=u8 255, "Modbus master in"=w459) -> ("error out"=w456:errorcluster, "Modbus master out"=w458:refnum<class "Modbus Master.lvclass">)  [unwired: 7 in]
            n154 = call-dynamic "Write Multiple Holding Registers.vi"("error in (no error)"=w456, "holding register values"=w461, "starting address"=w462, "Modbus master in"=w458) -> ("error out"=w463:errorcluster, "Modbus master out"=w464:refnum<class "Modbus Master.lvclass">)  [unwired: 6 in]
          }
        }
      }
      n155 = for {
        tunnel: w404 -> [w466] mode=indexing
        tunnel: w402 -> [w465] mode=indexing
        n156 = call-dynamic "Close.vi"("error in (no error)"=w466, "Modbus master in"=w465) -> ()  [unwired: 9 in, 1 out]
      }
    }
    frame Enabled {
    }
  }
  n157 = disable-structure shown="Enabled" {
    frame Disabled {
      n158 = To Long Integer(number=10.0) -> (32bit integer=w479:i32)
      n159 = Split Number(x=w479) -> (hi(x)=w478:u16, lo(x)=w477:u16)
      n160 = Build Array(w477, w478) -> (w476:u16[])
      n161 = call-poly <vilib>:"Create Master Instance.vi"("error in (no error)"=errorcluster {"status"=FALSE, "code"=0, "source"=""}, "port (502)"=u16 502, "address"="169.168.167.102") -> ("error out"=w475:errorcluster, "TCP master instance"=w484:refnum<class "Modbus Master.lvclass">)  [unwired: 7 in]
      n162 = for {
        tunnel: w476 -> [w491] mode=indexing
        tunnel: [w490] -> w472 mode=indexing
        tunnel: [w489] -> w474
        tunnel: w475 -> [w489]
        tunnel: u8 0 -> [w488]
        n163 = Type Cast(type=w488, x=w491) -> (*(type *) &x=w490:u8)
      }
      n164 = call-dynamic "Write Multiple Holding Registers.vi"("error in (no error)"=w474, "holding register values"=w472, "starting address"=u16 135, "Modbus master in"=w484) -> ("error out"=w482:errorcluster, "Modbus master out"=w483:refnum<class "Modbus Master.lvclass">)  [unwired: 6 in]
      n165 = call-dynamic "Close.vi"("error in (no error)"=w482, "Modbus master in"=w483) -> ()  [unwired: 9 in, 1 out]
    }
    frame Enabled {
    }
  }
